vi "Log to string array.vi"(10 "new line":string, 11 "Logg array in":string[](array[string])) -> (3 "Logg array out":string[](array[string]))   [LabVIEW 2017]
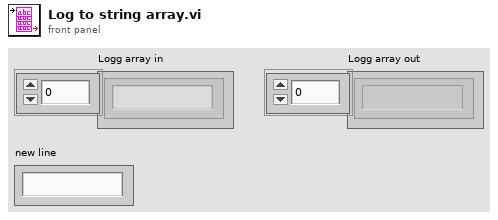
[diagram p1: front panel]
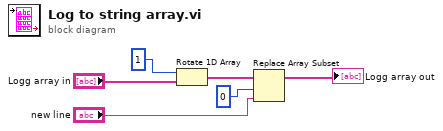
[diagram p0: block diagram]
diagram:
  n1 = Rotate 1D Array(1:"Logg array in", 2:1 ("n")) -> (0:w2:string[])
  n2 = Replace Array Subset(array=w2, new element="new line", index=0) -> (→"Logg array out":string[])
